vi "sv_Check Data Valid [Octave].vi"(0 "scaled signal [EU]":waveform(dbl), 1 "frequency range (1/1)":T7={"low band"=enum."16 Hz", "high band"=enum."16000 Hz"}, 3 "frequency range [Hz]":T6={"low frequency"=125.0, "high frequency"=8000.0} {"high frequency" min=0.001 format="%.2f"; "low frequency" min=0.001 format="%.2f"}, 4 "frequency range (1/3)":T2={"low band"=enum."20 Hz", "high band"=enum."20000 Hz"}, 5 "error in (no error)":errorcluster, 6 "restart averaging (F)":bool, 7 "bandwidth":enum16{"1/1", "1/3", "1/n"}(ring)=enum."1/n", 8 "reset filter (F)":bool, 9 "averaging type":T5(ring), 10 "1/n octave settings":T4={"standard"=enum."ANSI S1.11", "bandwidth"=enum."1/3 octave"}, 11 "exp avg settings":T1={" mode"=enum."Fast", "time constant [ms]"=125.0} {"time constant [ms]" format="%.2f"}, 13 "equal confidence level [dB]":dbl=1.0 format="%.2f") -> (14 "dup scaled signal [EU]":waveform(dbl), 15 "band number":cluster{"low band":i32, "high band":i32}, 17 "Restart averaging":bool, 18 "Reset Filter":bool, 19 "error out":errorcluster)   [LabVIEW 2017, in "SoundVib_Octave.lvlib"]
uses:
  <vilib>/addons/Sound and Vibration/svt_Octave/SoundVib_Octave.lvlib
  <vilib>/addons/_NISVFA/_Shared subVIs/Controls/svc_Octave Standard.ctl
  <vilib>/addons/_NISVFA/_Shared subVIs/Common/svc_Check for Waveform Parameter Continuity (no state).vi
  <vilib>/addons/_NISVFA/_Shared subVIs/Common/svc_Get SV Channel Info.vi
  <vilib>/addons/_NISVFA/_Shared subVIs/Common/svc_Engineering Units to Unit Label.vi
  <vilib>/addons/_NISVFA/_Shared subVIs/Common/svc_Unit Label to Engineering Units.vi
  <vilib>/addons/Sound and Vibration/svt_Octave_2014 standard/SoundVib_Octave_2014 standard.lvlib
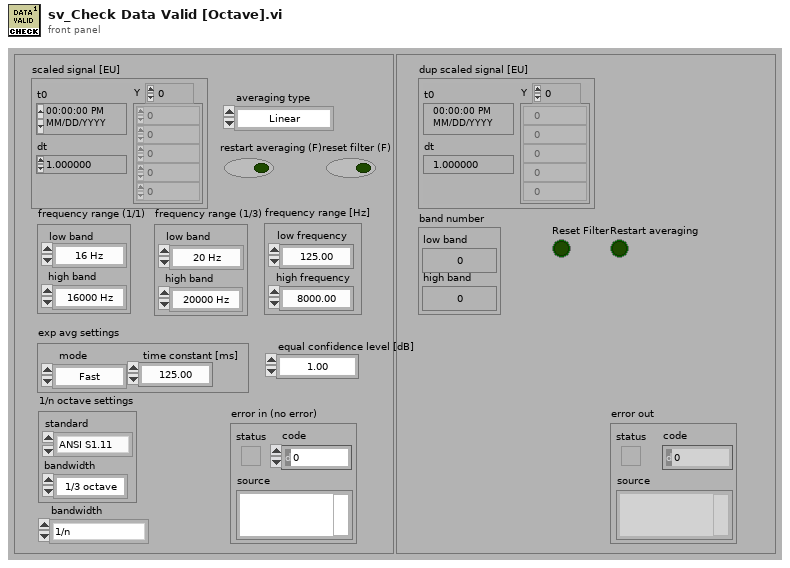
[diagram p1: front panel]
types:
  T1 = cluster{" mode":enum16{"Slow", "Fast", "Impulse", "Custom"}, "time constant [ms]":dbl}
  T2 = cluster{"low band":enum16{"20 Hz", "25 Hz", "31.5 Hz", "40 Hz", "50 Hz", "63 Hz", "80 Hz", "100 Hz", "125 Hz", "160 Hz", "200 Hz", "250 Hz", "315 Hz", "400 Hz", "500 Hz", "630 Hz", "800 Hz", "1000 Hz", "1250 Hz", "1600 Hz", "2000 Hz", "2500 Hz", "3150 Hz", "4000 Hz", "5000 Hz", "6300 Hz", "8000 Hz", "10000 Hz", "12500 Hz", "16000 Hz", "20000 Hz"}, "high band":enum16{"20 Hz", "25 Hz", "31.5 Hz", "40 Hz", "50 Hz", "63 Hz", "80 Hz", "100 Hz", "125 Hz", "160 Hz", "200 Hz", "250 Hz", "315 Hz", "400 Hz", "500 Hz", "630 Hz", "800 Hz", "1000 Hz", "1250 Hz", "1600 Hz", "2000 Hz", "2500 Hz", "3150 Hz", "4000 Hz", "5000 Hz", "6300 Hz", "8000 Hz", "10000 Hz", "12500 Hz", "16000 Hz", "20000 Hz"}}
  T3 = typedef "svc_Octave Standard.ctl" = enum16{"ANSI S1.11", "IEC 61260"}
  T4 = cluster{"standard":T3, "bandwidth":enum16{"1 octave", "1/3 octave", "1/6 octave", "1/12 octave", "1/24 octave"}}
  T5 = enum16{"Linear", "Exponential", "Equal confidence", "Peak"}
  T6 = cluster{"low frequency":dbl, "high frequency":dbl}
  T7 = cluster{"low band":enum16{"16 Hz", "31.5 Hz", "63 Hz", "125 Hz", "250 Hz", "500 Hz", "1000 Hz", "2000 Hz", "4000 Hz", "8000 Hz", "16000 Hz"}, "high band":enum16{"16 Hz", "31.5 Hz", "63 Hz", "125 Hz", "250 Hz", "500 Hz", "1000 Hz", "2000 Hz", "4000 Hz", "8000 Hz", "16000 Hz"}}
  T8 = cluster{"dt":bool, "t0 continuity":bool, "array length":bool, "channel info":bool, "name":bool}
  T9 = enum16{"1 octave", "1/3 octave", "1/6 octave", "1/12 octave", "1/24 octave", "1/48 octave", "1/96 octave"}
  T10 = enum16{"1 octave", "1/3 octave", "1/6 octave", "1/12 octave", "1/24 octave"}
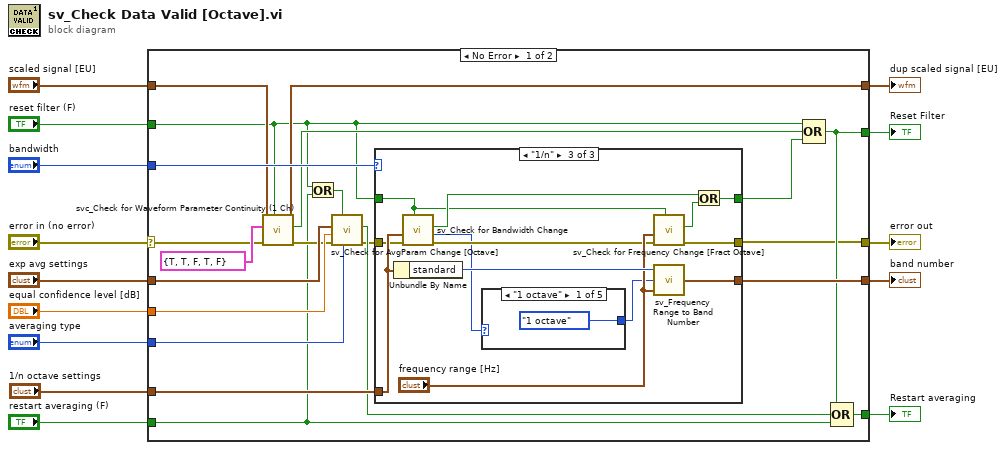
[diagram p0: block diagram]
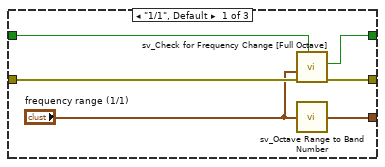
[diagram p2: hidden frame]
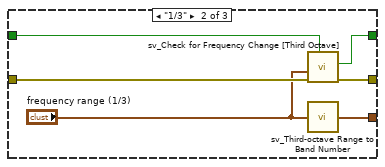
[diagram p3: hidden frame]
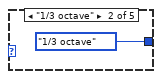
[diagram p4: hidden frame]
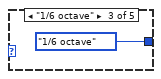
[diagram p5: hidden frame]
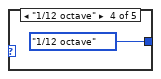
[diagram p6: hidden frame]
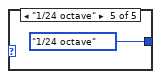
[diagram p7: hidden frame]
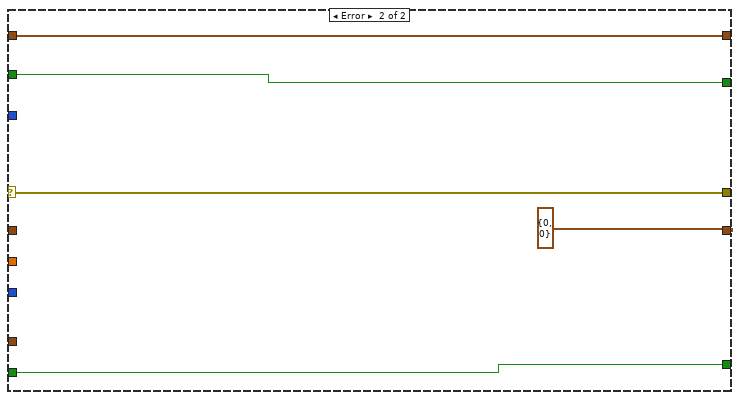
[diagram p8: hidden frame]
diagram:
  n1 = case shown="No Error" "error in (no error)" {
    selector: "error in (no error)" -> [w22 w67]
    tunnel: [w35 cluster{"low band":i32, "high band":i32} {"low band"=0, "high band"=0} ("band number")] -> w14
    tunnel: "exp avg settings" -> [w34 _]
    tunnel: "equal confidence level [dB]" -> [w33 _]
    tunnel: "averaging type" -> [w32 _]
    tunnel: [w18 w67] -> w10
    tunnel: [w27 w69] -> w9
    tunnel: "restart averaging (F)" -> [w16 w68]
    tunnel: "1/n octave settings" -> [w31 _]
    tunnel: "scaled signal [EU]" -> [w21 w66]
    tunnel: "reset filter (F)" -> [w17 w69]
    tunnel: [w26 w68] -> w5
    tunnel: "bandwidth" -> [w30 _]
    tunnel: [w20 w66] -> w1
    frame No Error {
      n2 = call <vilib>:"svc_Check for Waveform Parameter Continuity (1 Ch).vi"("restart averaging (F)"=w17, "error in (no error)"=w22, "checks for channel parameter change"=T8 {"dt"=TRUE, "t0 continuity"=TRUE, "array length"=FALSE, "channel info"=TRUE, "name"=FALSE}, "scaled signal [EU]"=w21) -> ("error out"=w25:errorcluster, "waveform parameter changed"=w23:bool, "dup scaled signal [EU]"=w20:waveform(dbl))  [unwired: 2 in, 3 out]
      n3 = Or(x=w17, y=w16) -> (x .or. y?=w15:bool)
      n4 = call <vilib>:"sv_Check for AvgParam Change [Octave].vi"("averaging type"=w32, "restart averaging (F) /reset"=w15, "error in (no error)"=w25, "equal confidence level [dB]"=w33, "exp avg settings"=w34) -> ("error out"=w19:errorcluster, "Param_has_changed"=w28:bool)  [unwired: 5 in]
      n5 = case shown="\"1/n\"" w30 {
        tunnel: [w41 w47 w60] -> w35
        tunnel: w19 -> [w40 w46 w55]
        tunnel: [w38 w45 w51] -> w18
        tunnel: w31 -> [_ _ w58]
        tunnel: [w37 w44 w52] -> w29
        tunnel: w17 -> [w36 w42 w50]
        frame "1/1", Default {
          n6 = call <vilib>:"sv_Check for Frequency Change [Full Octave].vi"("reset filter (F)"=w36, "error in (no error)"=w40, "frequency range (1/1)"="frequency range (1/1)") -> ("error out"=w38:errorcluster, "Param_has_changed"=w37:bool)  [unwired: 7 in]
          n7 = call <vilib>:"sv_Octave Range to Band Number.vi"("frequency range"="frequency range (1/1)") -> ("band number"=w41:cluster{"low band":i32, "high band":i32})
        }
        frame "1/3" {
          n8 = call <vilib>:"sv_Check for Frequency Change [Third Octave].vi"("reset filter (F)"=w42, "error in (no error)"=w46, "frequency range (1/3)"="frequency range (1/3)") -> ("error out"=w45:errorcluster, "Param_has_changed"=w44:bool)  [unwired: 7 in]
          n9 = call <vilib>:"sv_Third-octave Range to Band Number.vi"("frequency range"="frequency range (1/3)") -> ("band number"=w47:cluster{"low band":i32, "high band":i32})
        }
        frame "1/n" {
          n10 = Unbundle By Name(w58) -> ("standard"=w57:T3)
          n11 = call <vilib>:"sv_Check for Bandwidth Change.vi"("reset filter (F)"=w50, "error in (no error)"=w55, "1/n octave settings"=w58) -> ("error out"=w54:errorcluster, "bandwidth"=w49:T10, "parameter has changed"=w53:bool)  [unwired: 6 in]
          n12 = case shown="\"1 octave\"" w49 {
            tunnel: [T9."1 octave" ("bandwidth") T9."1/3 octave" ("bandwidth") T9."1/6 octave" ("bandwidth") T9."1/12 octave" ("bandwidth") T9."1/24 octave" ("bandwidth")] -> w48
            frame "1 octave" {
            }
            frame "1/3 octave" {
            }
            frame "1/6 octave" {
            }
            frame "1/12 octave" {
            }
            frame "1/24 octave" {
            }
          }
          n13 = call <vilib>:"sv_Check for Frequency Change [Fract Octave].vi"("reset filter (F)"=w50, "error in (no error)"=w54, "frequency range [Hz]"="frequency range [Hz]") -> ("error out"=w51:errorcluster, "Param_has_changed"=w59:bool)  [unwired: 7 in]
          n14 = call <vilib>:"sv_Frequency Range to Band Number.vi"("frequency range [Hz]"="frequency range [Hz]", "bandwidth"=w48, "standard"=w57) -> ("band number"=w60:cluster{"low band":i32, "high band":i32})
          n15 = Or(x=w53, y=w59) -> (x .or. y?=w52:bool)
        }
      }
      n16 = Compound Arithmetic op=OR(w17, w23, w29) -> (w27:bool)
      n17 = Compound Arithmetic op=OR(w27, w28, w16) -> (w26:bool)
    }
    frame Error {
    }
  }
  "dup scaled signal [EU]" <- w1
  "error out" <- w10
  "Reset Filter" <- w9
  "band number" <- w14
  "Restart averaging" <- w5
